vi "eFGV - MQTT Sub Unsub.vi"(6 "State":T2, 8 "error in (no error)":errorcluster, 10 "MQTT Sub Unsub":T1) -> (0 "error out":errorcluster, 2 "Event - MQTT Sub Unsub":refnum<user-event>)   [LabVIEW 2020]
uses:
  Control/State - eFGV.ctl
  Control/MQTT Sub Unsub.ctl
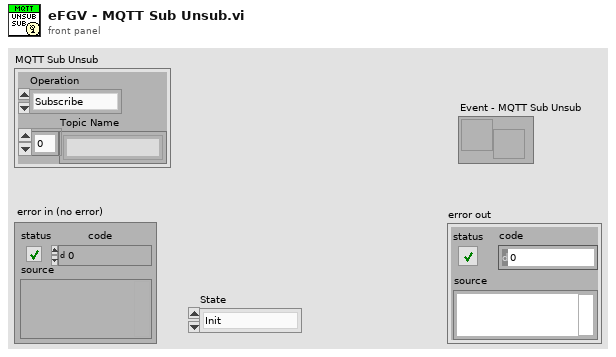
[diagram p1: front panel]
types:
  T1 = typedef "MQTT Sub Unsub.ctl" = cluster{"Operation":enum16{"Subscribe", "Unsubscribe"}, "Topic Name":string[]}
  T2 = typedef "State - eFGV.ctl" = enum16{"Init", "Read", "Write", "Close"}
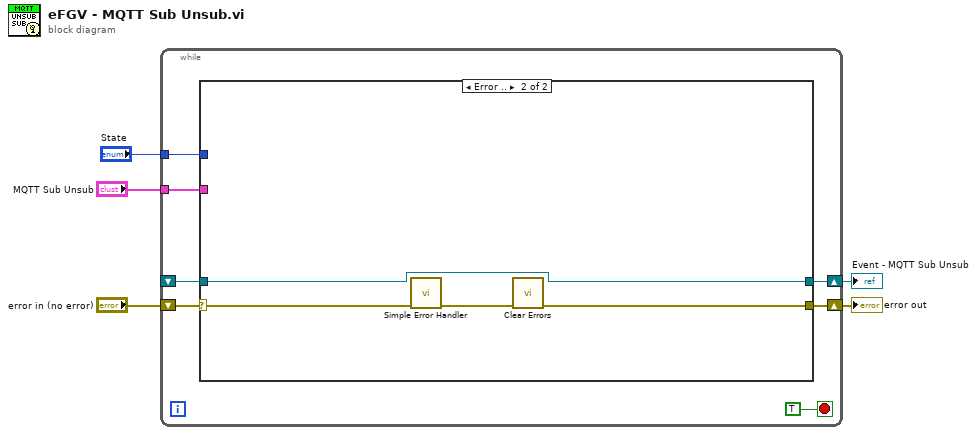
[diagram p0: block diagram]
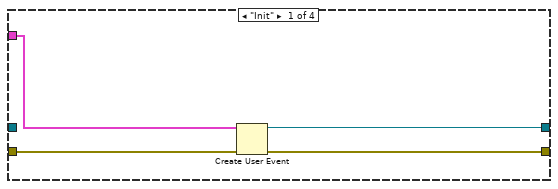
[diagram p3: hidden frame]
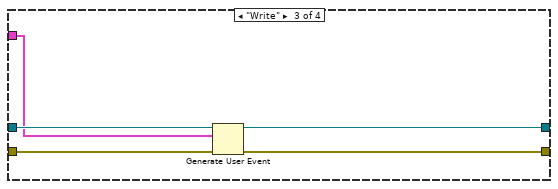
[diagram p4: hidden frame]
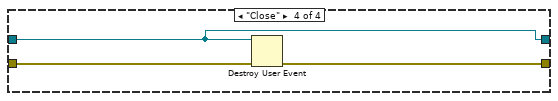
[diagram p5: hidden frame]
diagram:
  n1 = while {
    tunnel: "State" -> [w11]
    shift-right: [w9] -> w3
    shift-left: "error in (no error)" -> [w10]
    tunnel: "MQTT Sub Unsub" -> [w8]
    shift-right: [w7] -> w1
    shift-left: _ -> [w6]
    stop <- TRUE stop-if-true
    n2 = case shown="Error .." w10 {
      selector: w10 -> [w17 w36]
      tunnel: w11 -> [w18 _]
      tunnel: [w16 w34] -> w9
      tunnel: w8 -> [w15 _]
      tunnel: [w14 w33] -> w7
      tunnel: w6 -> [w13 w33]
      frame No Error {
        n3 = case shown="\"Read\", Default" w18 {
          tunnel: w17 -> [w22 w24 w29 w32]
          tunnel: [w21 w24 w28 w31] -> w16
          tunnel: w15 -> [w20 _ w26 _]
          tunnel: [w19 w23 w25 w30] -> w14
          tunnel: w13 -> [_ w23 w27 w30]
          frame "Init" {
            n4 = Create User Event(user event datatype=w20, error in=w22) -> (user event=w19:refnum<user-event>, error out=w21:errorcluster)
          }
          frame "Read", Default {
          }
          frame "Write" {
            n5 = Generate User Event(user event=w27, event data cluster=w26, error in=w29) -> (user event out=w25:refnum<user-event>, error out=w28:errorcluster)  [unwired: 1 in]
          }
          frame "Close" {
            n6 = Destroy User Event(user event=w30, error in=w32) -> (error out=w31:errorcluster)
          }
        }
      }
      frame Error {
        n7 = call <vilib>:"Simple Error Handler.vi"("error in (no error)"=w36) -> ("error out"=w35:errorcluster)  [unwired: 4 in, 4 out]
        n8 = call <vilib>:"Clear Errors.vi"("error in (no error)"=w35) -> ("error out"=w34:errorcluster)  [unwired: 5 in, 1 out]
      }
    }
  }
  "error out" <- w3
  "Event - MQTT Sub Unsub" <- w1
